vi "demo - auto-index tunnel for loop.vi"() -> ()   [LabVIEW 2024]
doc: "#vi_description \nPlot a finite sine wave onto a waveform graph\nThetic Engineering Ltd."
panel:
  out "current iteration":i32
  out "Waveform Graph":dbl[](graph)
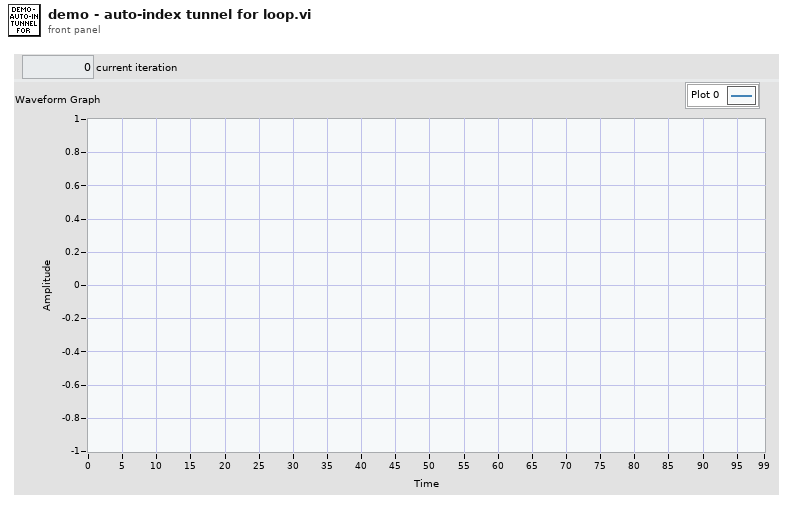
[diagram p1: front panel]
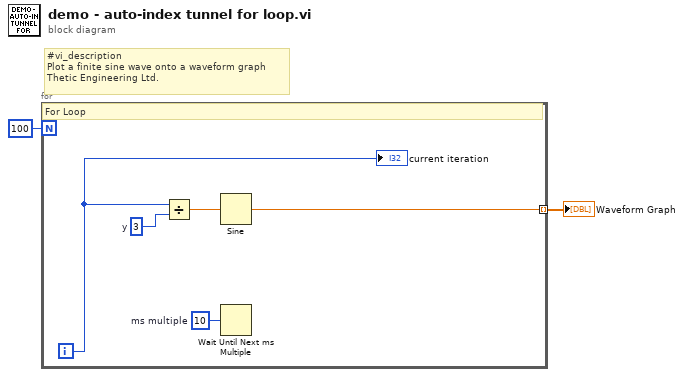
[diagram p0: block diagram]
diagram:
  # "#vi_description \nPlot a finite sine wave onto a waveform graph\nThetic Engineering Ltd."
  n1 = for {
    N: 100 -> [_]
    tunnel: [w3] -> w1 mode=indexing
    i -> [w4]
    w5 = u32 10  # ms multiple
    w6 = 3  # y
    # "For Loop"
    n2 = Divide(x=w4, y=w6) -> (x/y=w7:dbl)
    n3 = Sine(x=w7) -> (sin(x)=w3:dbl)
    n4 = Wait Until Next ms Multiple(millisecond multiple=w5) -> ()  [unwired: 1 out]
    "current iteration" <- w4
  }
  "Waveform Graph" <- w1
